vi "FT_Get_Modem_Status.vi"(0 "Handle":u32) -> (1 "FT_Status":u32, 2 "Modem Status":T1)   [LabVIEW 2011]
uses:
  FTD2XX.dll
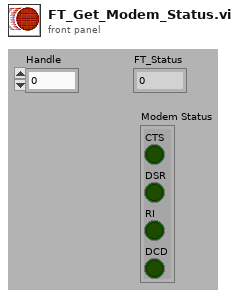
[diagram p1: front panel]
types:
  T1 = cluster{"CTS":bool, "DSR":bool, "RI":bool, "DCD":bool}
  T2 = cluster{"Boolean array[0]":bool, "Boolean array[1]":bool, "Boolean array[2]":bool, "Boolean array[3]":bool, "Boolean array[4]":bool, "Boolean array[5]":bool, "Boolean array[6]":bool, "Boolean array[7]":bool}
  T3 = cluster{"Boolean array[4]":bool, "Boolean array[5]":bool, "Boolean array[6]":bool, "Boolean array[7]":bool}
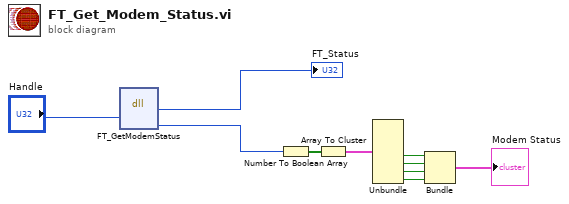
[diagram p0: block diagram]
diagram:
  n1 = dll-call lib="FTD2XX.dll" fn="FT_GetModemStatus"("Handle"="Handle") -> ("FT_Status"=→"FT_Status":u32, "ModemStatus"=w7:u32)  [unwired: 4 in, 3 out]
  n2 = Number To Boolean Array(number=w7) -> (Boolean array=w1:bool[])
  n3 = Array To Cluster(array=w1) -> (cluster=w6:T2)
  n4 = Unbundle(w6) -> ("Boolean array[4]"=w5:bool, "Boolean array[5]"=w4:bool, "Boolean array[6]"=w3:bool, "Boolean array[7]"=w2:bool)  [unwired: 4 out]
  n5 = Bundle("Boolean array[4]"=w5, "Boolean array[5]"=w4, "Boolean array[6]"=w3, "Boolean array[7]"=w2) -> (→"Modem Status":T3)  [unwired: 1 out]
